vi "TestMove.vi"() -> ()   [LabVIEW 2017]
uses:
  <vilib>/userdefined/High Color/IMAQdx.ctl
  Global 5.vi
  <vilib>/vision/NI_Vision_Development_Module.lvlib
  <vilib>/vision/driver/NI_Vision_Acquisition_Software.lvlib
panel:
  out "x-y":dbl
  out "Back":bool
  out "ROI 2":T1
  out "Im3":T2(plugin-control)
  out "SecondCount":T2(plugin-control)
  out "Number of Objects 3":i32
  out "Less?":bool
  out "Encode Back":dbl
  out "Count Encode":dbl
  out "Status":string
  out "ROI":T1
  out "Count":T2(plugin-control)
  out "Extract":T2(plugin-control)
  out "Particle":T2(plugin-control)
  out "Threshold":T2(plugin-control)
  in  "Settings":T3={"Objects"=0, "Threshold"=128, "Reject Border"=FALSE, "Fill Holes"=FALSE, "Min Object Size"=FALSE, "Min Size"=3, "Max Object Size"=FALSE, "Max Size"=100, "Show Search Area"=FALSE, "Show Center"=TRUE, "Show Bounding Box"=TRUE} {"Objects" items=["Bright Objects", "Dark Objects"]; "Threshold" min=1 max=999999999 step=1; "Max Size" min=1 max=999999999 step=1; "Min Size" min=1 max=999999999 step=1}
  in  "Number of Objects":i32
  out "Number of Objects 2":i32
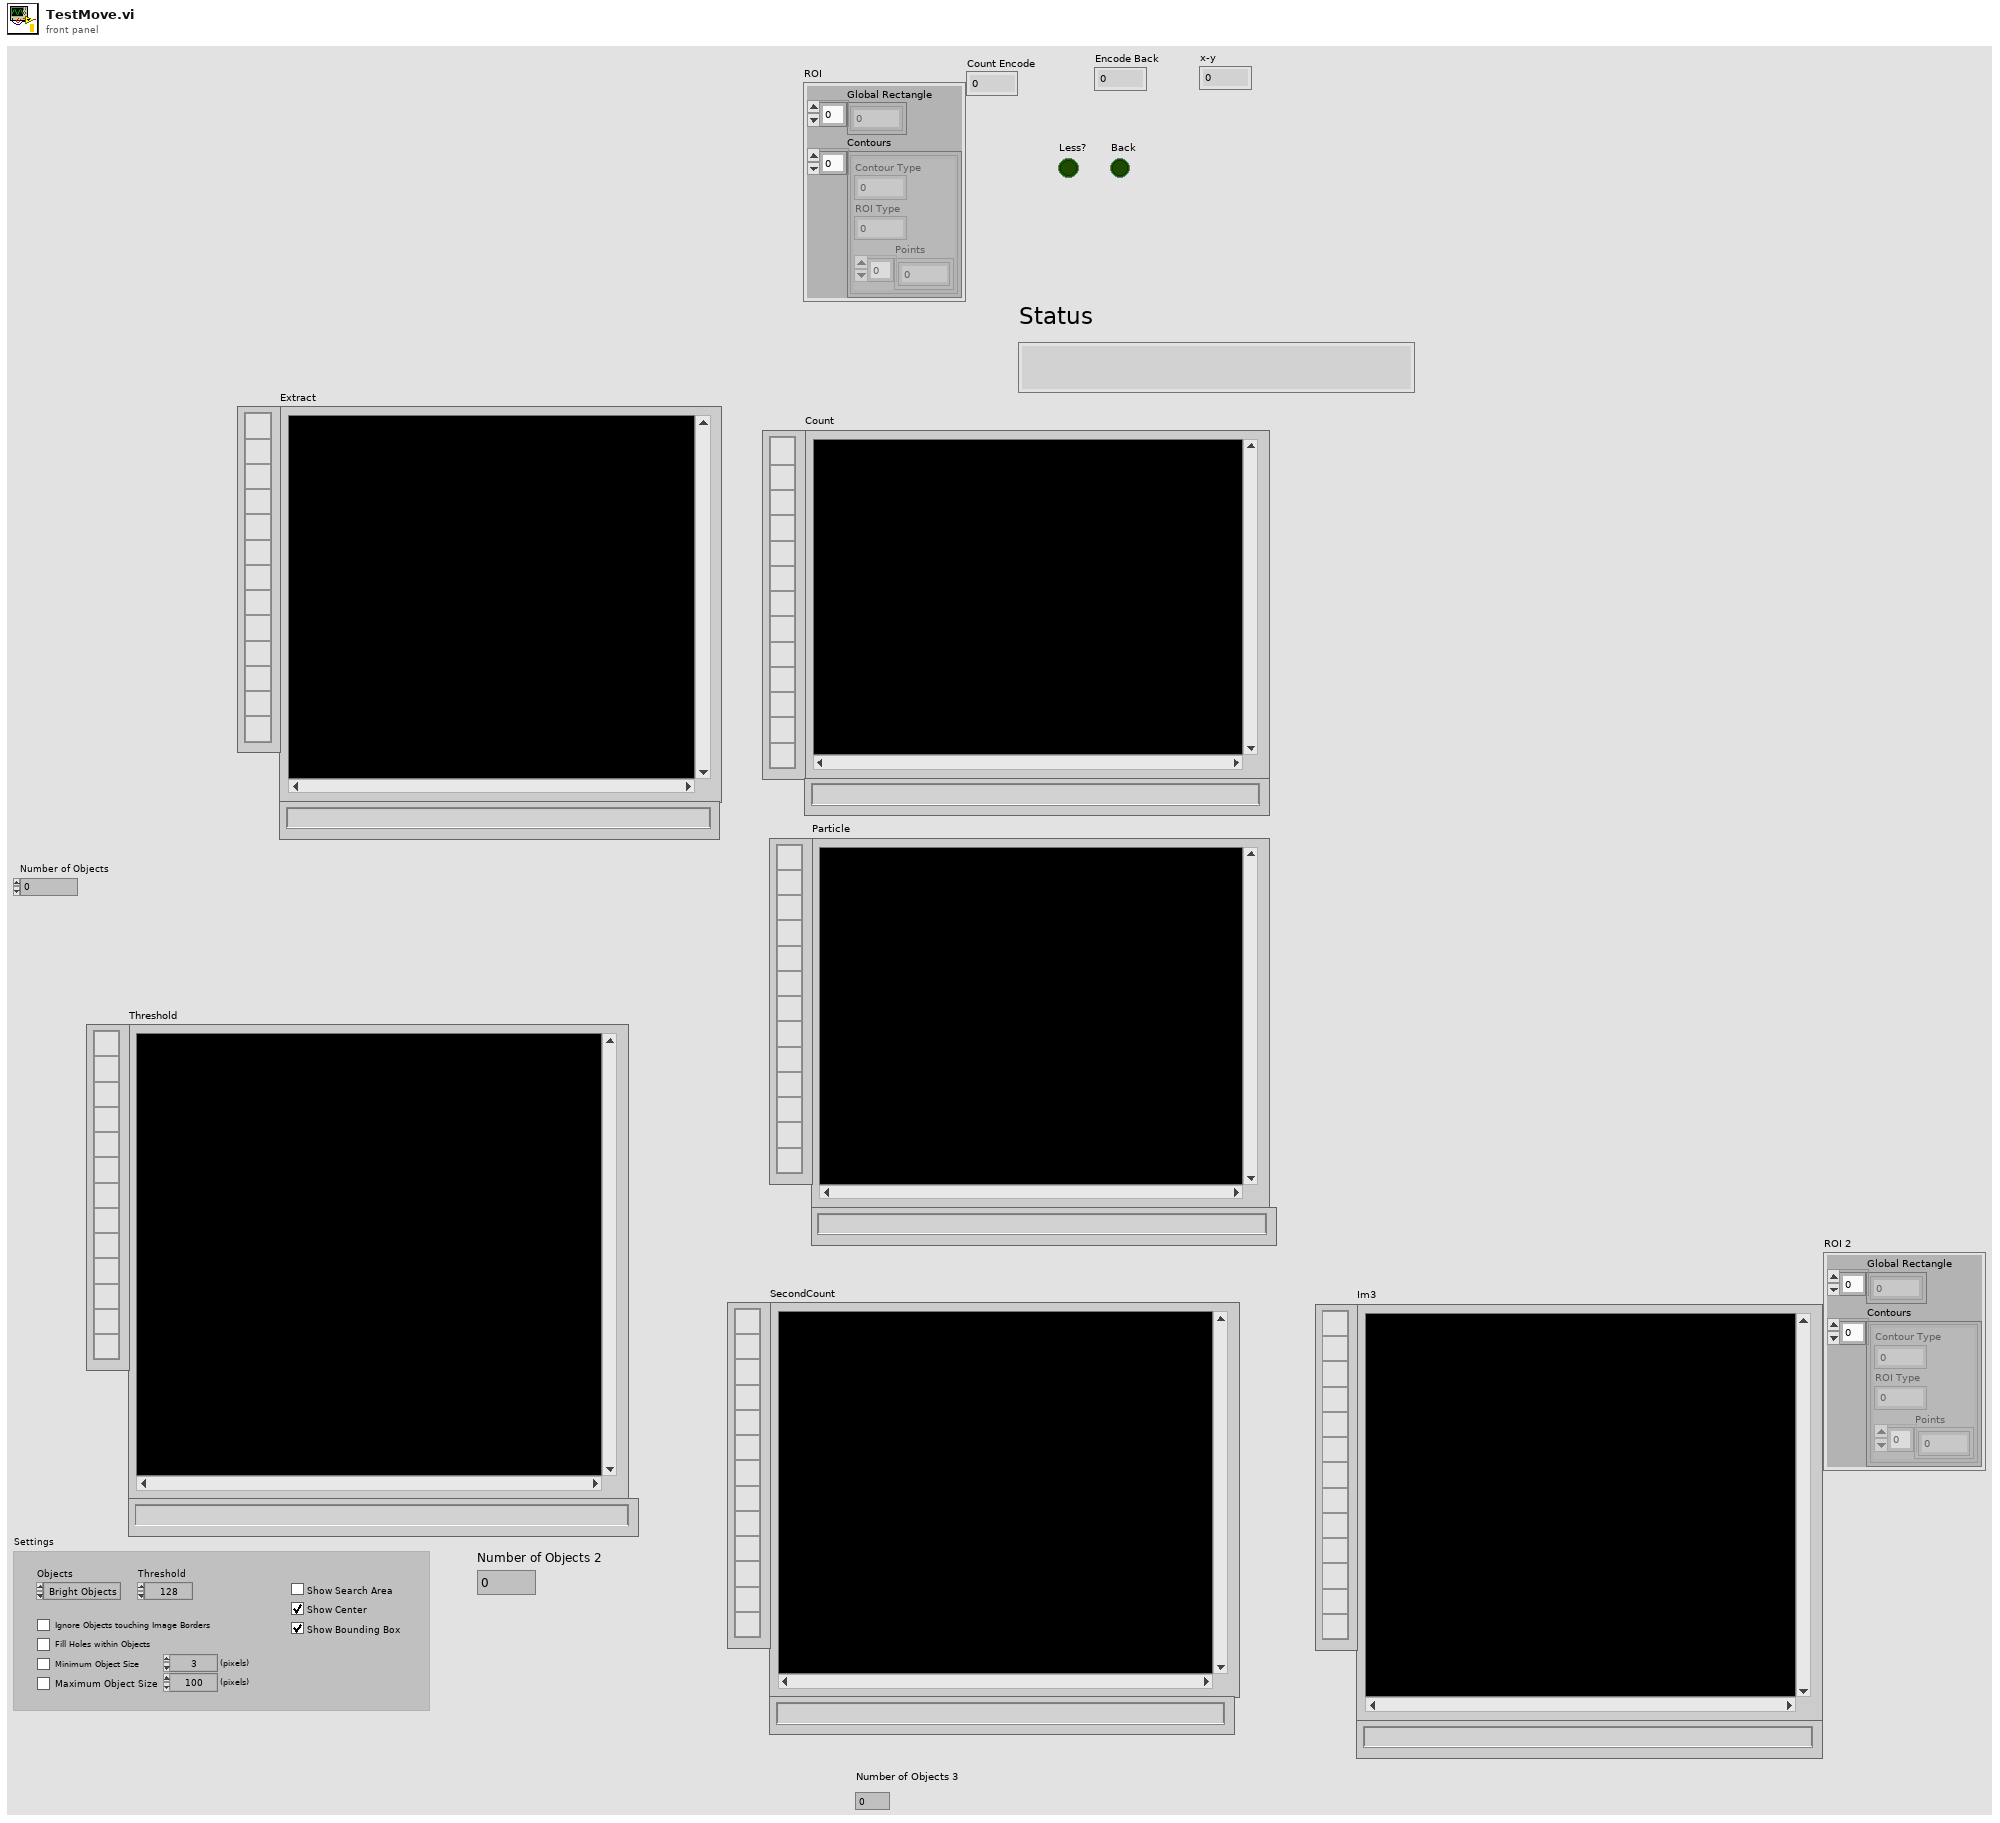
[diagram p1: front panel]
types:
  T1 = cluster{"Global Rectangle":i32[], "Contours":cluster{"Contour Type":u32, "ROI Type":u32, "Points":i32[]}[]}
  T2 = typedef "IMAQ Image.ctl" = refnum<image>
  T3 = cluster{"Objects":u16, "Threshold":i32, "Reject Border":bool, "Fill Holes":bool, "Min Object Size":bool, "Min Size":i32, "Max Object Size":bool, "Max Size":i32, "Show Search Area":bool, "Show Center":bool, "Show Bounding Box":bool}
  T4 = typedef "IMAQdx.ctl" = refnum<k21>
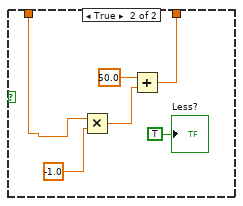
[diagram p2: hidden frame]
diagram:
  n1 = flat-sequence {
    tunnel: [w140] -> w90
    tunnel: [w139] -> w89
    tunnel: [w136] -> w88
    tunnel: [w151] -> w121
    tunnel: [w150] -> w120
    tunnel: w90 -> [w151]
    tunnel: w89 -> [w150]
    tunnel: w88 -> [w149]
    tunnel: [w148] -> w87
    tunnel: w121 -> [w160]
    tunnel: w120 -> [w159]
    tunnel: [w160] -> w115
    tunnel: [w159] -> w114
    tunnel: w87 -> [w158]
    tunnel: [w157] -> w86
    tunnel: [w170] -> w117
    tunnel: [w169] -> w116
    tunnel: w115 -> [w170]
    tunnel: w114 -> [w169]
    tunnel: w86 -> [w166]
    tunnel: [w164] -> w85
    tunnel: w117 -> [w179]
    tunnel: w116 -> [w178]
    tunnel: [w179] -> w103
    tunnel: [w178] -> w105
    tunnel: w85 -> [w177]
    tunnel: [w176] -> w83
    tunnel: w105 -> [w186]
    tunnel: [w186] -> w104
    tunnel: w103 -> [w185]
    tunnel: [w185] -> w102
    tunnel: [w183] -> w84
    tunnel: w83 -> [w183]
    tunnel: w104 -> [w193]
    tunnel: w102 -> [w192]
    tunnel: [w193] -> w119
    tunnel: [w192] -> w118
    tunnel: w84 -> [w189]
    tunnel: [w187] -> w82
    tunnel: w119 -> [w201]
    tunnel: w118 -> [w202]
    tunnel: [w202] -> w112
    tunnel: [w201] -> w110
    tunnel: w82 -> [w200]
    tunnel: [w199] -> w80
    tunnel: [w209] -> w113
    tunnel: w112 -> [w209]
    tunnel: [w208] -> w111
    tunnel: w110 -> [w208]
    tunnel: [w206] -> w81
    tunnel: w80 -> [w206]
    tunnel: [w212] -> w129
    tunnel: [w214] -> w128
    tunnel: w113 -> [w214]
    tunnel: w111 -> [w212]
    tunnel: w81 -> [w211]
    tunnel: [w210] -> w79
    tunnel: w129 -> [w223]
    tunnel: w128 -> [w224]
    tunnel: [w224] -> w109
    tunnel: [w223] -> w108
    tunnel: w79 -> [w222]
    tunnel: [w221] -> w78
    tunnel: [w232] -> w130
    tunnel: [w233] -> w127
    tunnel: w109 -> [w233]
    tunnel: w108 -> [w232]
    tunnel: w78 -> [w230]
    tunnel: [w228] -> w77
    tunnel: w130 -> [w240]
    tunnel: w127 -> [w241]
    tunnel: [w240] -> w56
    tunnel: w77 -> [w243]
    tunnel: [w242] -> w55
    tunnel: [w241] -> w54
    tunnel: [w240] -> w53
    tunnel: w56 -> [w253]
    tunnel: [w249] -> w107
    tunnel: [w253] -> w106
    tunnel: [w247] -> w76
    tunnel: w55 -> [w250]
    tunnel: w54 -> [w249]
    tunnel: w53 -> [w248]
    tunnel: [w308] -> w131
    tunnel: [w309] -> w126
    tunnel: w107 -> [w309]
    tunnel: w106 -> [w308]
    tunnel: w76 -> [w306]
    tunnel: [w304] -> w75
    tunnel: w131 -> [w319]
    tunnel: w126 -> [w318]
    tunnel: [w318] -> w101
    tunnel: [w319] -> w100
    tunnel: [w318] -> w99
    tunnel: w75 -> [w317]
    tunnel: [w316] -> w74
    tunnel: w101 -> [_]
    tunnel: w100 -> [w325]
    tunnel: [w325] -> w65
    tunnel: [w324] -> w64
    tunnel: w99 -> [w324]
    tunnel: w74 -> [w323]
    tunnel: [w323] -> w63
    tunnel: w65 -> [w331]
    tunnel: w64 -> [w332]
    tunnel: [w332] -> w94
    tunnel: [w331] -> w92
    tunnel: w63 -> [w329]
    tunnel: [w327] -> w73
    tunnel: w94 -> [w343]
    tunnel: [w343] -> w93
    tunnel: w92 -> [w344]
    tunnel: [w344] -> w91
    tunnel: w73 -> [w342]
    tunnel: [w341] -> w72
    tunnel: w93 -> [w356]
    tunnel: [w356] -> w98
    tunnel: w91 -> [w357]
    tunnel: [w357] -> w96
    tunnel: w72 -> [w354]
    tunnel: [w352] -> w71
    tunnel: w98 -> [w376]
    tunnel: [w376] -> w97
    tunnel: w96 -> [w375]
    tunnel: [w375] -> w95
    tunnel: w71 -> [w374]
    tunnel: [w373] -> w70
    tunnel: [w383] -> w125
    tunnel: [w384] -> w132
    tunnel: w97 -> [w384]
    tunnel: w95 -> [w383]
    tunnel: w70 -> [w382]
    tunnel: [w380] -> w69
    tunnel: w125 -> [w395]
    tunnel: [w395] -> w124
    tunnel: w132 -> [w394]
    tunnel: [w394] -> w133
    tunnel: w69 -> [w393]
    tunnel: [w392] -> w68
    tunnel: w124 -> [w403]
    tunnel: w133 -> [w404]
    tunnel: [w403] -> w123
    tunnel: [w404] -> w134
    tunnel: w68 -> [w401]
    tunnel: [w399] -> w67
    tunnel: w123 -> [w413]
    tunnel: w134 -> [w414]
    tunnel: [w414] -> w52
    tunnel: [w413] -> w50
    tunnel: w67 -> [w412]
    tunnel: [w411] -> w48
    tunnel: w52 -> [w420]
    tunnel: [w420] -> w51
    tunnel: w50 -> [w419]
    tunnel: [w419] -> w49
    tunnel: w48 -> [w418]
    tunnel: [w418] -> w47
    tunnel: [w426] -> w122
    tunnel: [w427] -> w135
    tunnel: w51 -> [w427]
    tunnel: w49 -> [w426]
    tunnel: w47 -> [w424]
    tunnel: [w422] -> w66
    tunnel: w122 -> [w432]
    tunnel: w135 -> [w433]
    tunnel: w66 -> [w435]
    tunnel: [w434] -> w44
    tunnel: [w433] -> w45
    tunnel: [w432] -> w46
    tunnel: [w442] -> w62
    tunnel: w46 -> [w442]
    tunnel: [w441] -> w61
    tunnel: w45 -> [w441]
    tunnel: [w440] -> w60
    tunnel: w44 -> [w440]
    tunnel: [w446] -> w59
    tunnel: w62 -> [w446]
    tunnel: [w445] -> w58
    tunnel: w61 -> [w445]
    tunnel: w60 -> [w449]
    tunnel: [w444] -> w57
    tunnel: w59 -> [w455]
    tunnel: w58 -> [w456]
    tunnel: w57 -> [w458]
    tunnel: [w457] -> w43
    tunnel: [w456] -> w42
    tunnel: [w455] -> w41
    tunnel: w43 -> [w465]
    tunnel: w42 -> [w463]
    tunnel: w41 -> [w462]
    tunnel: [w462] -> w40
    tunnel: [w464] -> w39
    tunnel: [w463] -> w37
    tunnel: [w462] -> w36
    tunnel: w40 -> [w479]
    tunnel: w39 -> [w478]
    tunnel: [w477] -> w38
    tunnel: w37 -> [w477]
    tunnel: w36 -> [w476]
    tunnel: [w476] -> w35
    tunnel: [w475] -> w31
    tunnel: w38 -> [w488]
    tunnel: w35 -> [w487]
    tunnel: [w486] -> w34
    tunnel: [w485] -> w33
    tunnel: [w484] -> w32
    tunnel: w31 -> [w483]
    tunnel: w34 -> [w540]
    tunnel: w33 -> [w538]
    tunnel: w32 -> [w537]
    tunnel: [w539] -> w30
    tunnel: [w538] -> w29
    tunnel: [w537] -> w28
    tunnel: w30 -> [w552]
    tunnel: w29 -> [w550]
    tunnel: w28 -> [w551]
    tunnel: [w551] -> w27
    tunnel: [w550] -> w25
    tunnel: [w549] -> w22
    tunnel: w27 -> [w559]
    tunnel: [w559] -> w26
    tunnel: w25 -> [w558]
    tunnel: [w558] -> w24
    tunnel: [w556] -> w23
    tunnel: w22 -> [w556]
    tunnel: w26 -> [w564]
    tunnel: w24 -> [w563]
    tunnel: w23 -> [w566]
    tunnel: [w562] -> w21
    tunnel: [w564] -> w20
    tunnel: [w563] -> w19
    tunnel: w21 -> [w577]
    tunnel: w20 -> [w576]
    tunnel: w19 -> [w575]
    tunnel: [w576] -> w18
    tunnel: [w575] -> w17
    tunnel: [w574] -> w16
    tunnel: w18 -> [w583]
    tunnel: w17 -> [w582]
    tunnel: w16 -> [w588]
    tunnel: [w584] -> w15
    tunnel: [w583] -> w13
    tunnel: [w582] -> w11
    tunnel: w15 -> [w597]
    tunnel: [w596] -> w14
    tunnel: w13 -> [w595]
    tunnel: [w595] -> w12
    tunnel: w11 -> [w594]
    tunnel: [w594] -> w10
    tunnel: w14 -> [w602]
    tunnel: w12 -> [w604]
    tunnel: w10 -> [w603]
    tunnel: [w604] -> w9
    tunnel: [w603] -> w7
    tunnel: [w602] -> w5
    tunnel: w9 -> [w615]
    tunnel: [w615] -> w8
    tunnel: w7 -> [w614]
    tunnel: [w614] -> w6
    tunnel: w5 -> [w613]
    tunnel: [w612] -> w4
    tunnel: w8 -> [w621]
    tunnel: w6 -> [w620]
    tunnel: w4 -> [w623]
    tunnel: [w621] -> w3
    tunnel: [w620] -> w2
    tunnel: [w619] -> w1
    tunnel: w3 -> [w633]
    tunnel: w2 -> [w632]
    tunnel: w1 -> [w631]
    frame #0 {
      w140 = tag "B/I2C" ("myRIO MXP Port A/B")
      w139 = u8 1 ("Controller ID#  (I2C Address)")
      # "enable"
      n2 = Wait (ms)(milliseconds to wait=u32 1000) -> ()  [unwired: 1 out]
      n3 = local write "Status"("Starting" ("Status")) -> ()
      n4 = call <vilib>:"TETRIX_Enable_DC_Controller_myRIO.vi"("myRIO MXP Port A/B"=w140, "Controller ID#  (I2C Address)"=w139) -> ("Error/Flow Out"=w138:errorcluster)  [unwired: 5 in]
      n5 = call <vilib>:"TETRIX_Motor_Invert_myRIO.vi"("myRIO MXP Port A/B"=w140, "Invert State"=TRUE, "Select Channel"="Motor 1", "Controller ID#  (I2C Address)"=w139) -> ()  [unwired: 3 in, 1 out]
      n6 = call <vilib>:"TETRIX_Reset_Encoders_myRIO.vi"("myRIO MXP Port A/B"=w140, "Select Encoder"="Encoders 1 and 2", "Controller ID#  (I2C Address)"=w139, "Error/Flow In"=w138) -> ("Error/Flow Out"=w137:errorcluster)  [unwired: 3 in]
      n7 = call <vilib>:"TETRIX_Stop_Motors_myRIO.vi"("myRIO MXP Port A/B"=w140, "Stop Mode"="Brake", "Select Channel"="Both Motors", "Controller ID#  (I2C Address)"=w139, "Error/Flow In"=w137) -> ("Error/Flow Out"=w136:errorcluster)  [unwired: 2 in]
    }
    frame #1 {
      w153 = 660 ("Motor 2 Encoder Target")
      w155 = i16 200 ("Motor 1 Contant Speed (Degrees per Second)")
      # "fate 1 start position"
      n8 = Wait (ms)(milliseconds to wait=u32 5500) -> ()  [unwired: 1 out]
      n9 = call <vilib>:"TETRIX_Set_Motor_Target(s)_myRIO.vi"("Motor 2 Encoder Target"=w153, "Motor 1 Encoder Target"=w153, "myRIO MXP Port A/B"=w151, "Controller ID#  (I2C Address)"=w150, "Motor 2 Constant Speed (Degrees per Second)"=w155, "Motor 1 Contant Speed (Degrees per Second)"=w155, "Encoder Units"="Degrees", "Error/Flow In"=w149) -> ("Error/Flow Out"=w148:errorcluster)  [unwired: 1 in]
      "Status" <- "Phase 1" ("Status")
    }
    frame #2 {
      n10 = Wait (ms)(milliseconds to wait=u32 500) -> ()  [unwired: 1 out]
      n11 = call <vilib>:"TETRIX_Stop_Motors_myRIO.vi"("myRIO MXP Port A/B"=w160, "Stop Mode"="Brake", "Select Channel"="Both Motors", "Controller ID#  (I2C Address)"=w159, "Error/Flow In"=w158) -> ("Error/Flow Out"=w157:errorcluster)  [unwired: 2 in]
    }
    frame #3 {
      w175 = i16 100 ("Motor 1 Contant Speed (Degrees per Second)")
      # "fate 2 catch ball"
      n12 = Wait (ms)(milliseconds to wait=u32 3000) -> ()  [unwired: 1 out]
      n13 = local write "Status"("Turning" ("Status")) -> ()
      n14 = call <vilib>:"TETRIX_Reset_Encoders_myRIO.vi"("myRIO MXP Port A/B"=w170, "Select Encoder"="Encoders 1 and 2", "Controller ID#  (I2C Address)"=w169, "Error/Flow In"=w166) -> ("Error/Flow Out"=w165:errorcluster)  [unwired: 3 in]
      n15 = call <vilib>:"TETRIX_Set_Motor_Target(s)_myRIO.vi"("Motor 2 Encoder Target"=300 ("Motor 1 Encoder Target"), "Motor 1 Encoder Target"=-290, "myRIO MXP Port A/B"=w170, "Controller ID#  (I2C Address)"=w169, "Motor 2 Constant Speed (Degrees per Second)"=w175, "Motor 1 Contant Speed (Degrees per Second)"=w175, "Encoder Units"="Degrees", "Error/Flow In"=w165) -> ("Error/Flow Out"=w164:errorcluster)  [unwired: 1 in]
    }
    frame #4 {
      n16 = Wait (ms)(milliseconds to wait=u32 500) -> ()  [unwired: 1 out]
      n17 = call <vilib>:"TETRIX_Stop_Motors_myRIO.vi"("myRIO MXP Port A/B"=w179, "Stop Mode"="Brake", "Select Channel"="Both Motors", "Controller ID#  (I2C Address)"=w178, "Error/Flow In"=w177) -> ("Error/Flow Out"=w176:errorcluster)  [unwired: 2 in]
    }
    frame #5 {
      n18 = local write "Status"("Move Gripper" ("Status")) -> ()
      n19 = call "ServoPickup.vi"() -> ()  [unwired: 12 in]
    }
    frame #6 {
      w195 = i16 100 ("Motor 1 Contant Speed (Degrees per Second)")
      n20 = Wait (ms)(milliseconds to wait=u32 5000) -> ()  [unwired: 1 out]
      n21 = local write "Status"("Moving to catch" ("Status")) -> ()
      n22 = call <vilib>:"TETRIX_Reset_Encoders_myRIO.vi"("myRIO MXP Port A/B"=w192, "Select Encoder"="Encoders 1 and 2", "Controller ID#  (I2C Address)"=w193, "Error/Flow In"=w189) -> ("Error/Flow Out"=w188:errorcluster)  [unwired: 3 in]
      n23 = call <vilib>:"TETRIX_Set_Motor_Target(s)_myRIO.vi"("Motor 2 Encoder Target"=390 ("Motor 1 Encoder Target"), "Motor 1 Encoder Target"=390, "myRIO MXP Port A/B"=w192, "Controller ID#  (I2C Address)"=w193, "Motor 2 Constant Speed (Degrees per Second)"=w195, "Motor 1 Contant Speed (Degrees per Second)"=w195, "Encoder Units"="Degrees", "Error/Flow In"=w188) -> ("Error/Flow Out"=w187:errorcluster)  [unwired: 1 in]
    }
    frame #7 {
      n24 = Wait (ms)(milliseconds to wait=u32 500) -> ()  [unwired: 1 out]
      n25 = call <vilib>:"TETRIX_Stop_Motors_myRIO.vi"("myRIO MXP Port A/B"=w202, "Stop Mode"="Brake", "Select Channel"="Both Motors", "Controller ID#  (I2C Address)"=w201, "Error/Flow In"=w200) -> ("Error/Flow Out"=w199:errorcluster)  [unwired: 2 in]
    }
    frame #8 {
      n26 = local write "Status"("Catching" ("Status")) -> ()
      n27 = call "PickBall.vi"() -> ()  [unwired: 12 in]
    }
    frame #9 {
      w217 = i16 100 ("Motor 1 Contant Speed (Degrees per Second)")
      n28 = Wait (ms)(milliseconds to wait=u32 4200) -> ()  [unwired: 1 out]
      n29 = call <vilib>:"TETRIX_Set_Motor_Target(s)_myRIO.vi"("Motor 2 Encoder Target"=390 ("Motor 1 Encoder Target"), "Motor 1 Encoder Target"=390, "myRIO MXP Port A/B"=w214, "Controller ID#  (I2C Address)"=w212, "Motor 2 Constant Speed (Degrees per Second)"=w217, "Motor 1 Contant Speed (Degrees per Second)"=w217, "Encoder Units"="Degrees", "Error/Flow In"=w211) -> ("Error/Flow Out"=w210:errorcluster)  [unwired: 1 in]
      n30 = local write "Status"("Moving to Bowling" ("Status")) -> ()
      n31 = call <vilib>:"TETRIX_Reset_Encoders_myRIO.vi"("myRIO MXP Port A/B"=w214, "Select Encoder"="Encoders 1 and 2", "Controller ID#  (I2C Address)"=w212) -> ()  [unwired: 4 in, 1 out]
    }
    frame #10 {
      # "end fate2"
      n32 = Wait (ms)(milliseconds to wait=u32 500) -> ()  [unwired: 1 out]
      n33 = call <vilib>:"TETRIX_Stop_Motors_myRIO.vi"("myRIO MXP Port A/B"=w224, "Stop Mode"="Brake", "Select Channel"="Both Motors", "Controller ID#  (I2C Address)"=w223, "Error/Flow In"=w222) -> ("Error/Flow Out"=w221:errorcluster)  [unwired: 2 in]
    }
    frame #11 {
      w237 = i16 100 ("Motor 2 Constant Speed (Degrees per Second)")
      # "fate 3  go to shoot ball position"
      n34 = Wait (ms)(milliseconds to wait=u32 3000) -> ()  [unwired: 1 out]
      n35 = local write "Status"("Phase 3 Turning" ("Status")) -> ()
      n36 = call <vilib>:"TETRIX_Reset_Encoders_myRIO.vi"("myRIO MXP Port A/B"=w233, "Select Encoder"="Encoders 1 and 2", "Controller ID#  (I2C Address)"=w232, "Error/Flow In"=w230) -> ("Error/Flow Out"=w229:errorcluster)  [unwired: 3 in]
      n37 = call <vilib>:"TETRIX_Set_Motor_Target(s)_myRIO.vi"("Motor 2 Encoder Target"=300, "Motor 1 Encoder Target"=-295, "myRIO MXP Port A/B"=w233, "Controller ID#  (I2C Address)"=w232, "Motor 2 Constant Speed (Degrees per Second)"=w237, "Motor 1 Contant Speed (Degrees per Second)"=w237, "Encoder Units"="Degrees", "Error/Flow In"=w229) -> ("Error/Flow Out"=w228:errorcluster)  [unwired: 1 in]
    }
    frame #12 {
      n38 = Wait (ms)(milliseconds to wait=u32 500) -> ()  [unwired: 1 out]
      n39 = call <vilib>:"TETRIX_Stop_Motors_myRIO.vi"("myRIO MXP Port A/B"=w241, "Stop Mode"="Brake", "Select Channel"="Both Motors", "Controller ID#  (I2C Address)"=w240, "Error/Flow In"=w243) -> ("Error/Flow Out"=w242:errorcluster)  [unwired: 2 in]
    }
    frame #13 {
      (unwired) "im0" ("Image Name")
      n40 = global write "Global 5.vi" "Count Encode"(0.0 ("Count Encode")) -> ()
      n41 = call "IMAQ Create"("Image Name"="im0") -> ("New Image"=w256:T2)  [unwired: 4 in, 1 out]
      n42 = call "IMAQ Create"("Image Name"="im1") -> ("New Image"=w254:T2)  [unwired: 4 in, 1 out]
      n43 = while {
        tunnel: w256 -> [w282]
        tunnel: w254 -> [w279]
        tunnel: w249 -> [w274]
        tunnel: w248 -> [w275]
        tunnel: w250 -> [w262]
        tunnel: w249 -> [w260]
        tunnel: w248 -> [w259]
        tunnel: [w258] -> w247
        stop <- w272 stop-if-true
        w283 = u16 1 items=["RGB", "HSL", "HSV", "HSI"] ("Color Mode")
        n44 = flat-sequence {
          tunnel: w275 -> [w296]
          tunnel: w274 -> [w295]
          tunnel: w262 -> [w287]
          tunnel: [w285] -> w261
          tunnel: w261 -> [w298]
          tunnel: w260 -> [w302]
          tunnel: w259 -> [w299]
          tunnel: [w297] -> w258
          frame #0 {
            w288 = 50 ("Motor 1 Encoder Target")
            w292 = i16 100 ("Motor 1 Contant Speed (Degrees per Second)")
            n45 = global read "Global 5.vi" "Count Encode"() -> (w289:dbl)
            n46 = Wait (ms)(milliseconds to wait=u32 500 ("millisecond timer value")) -> ()  [unwired: 1 out]
            n47 = Add(x=w288, y=w289) -> (x+y=w290:dbl)
            n48 = call <vilib>:"TETRIX_Reset_Encoders_myRIO.vi"("myRIO MXP Port A/B"=w295, "Select Encoder"="Encoders 1 and 2", "Controller ID#  (I2C Address)"=w296, "Error/Flow In"=w287) -> ("Error/Flow Out"=w286:errorcluster)  [unwired: 3 in]
            n49 = call <vilib>:"TETRIX_Set_Motor_Target(s)_myRIO.vi"("Motor 2 Encoder Target"=w288, "Motor 1 Encoder Target"=w288, "myRIO MXP Port A/B"=w295, "Motor 2 Constant Speed (Degrees per Second)"=w292, "Motor 1 Contant Speed (Degrees per Second)"=w292, "Encoder Units"="Degrees", "Error/Flow In"=w286) -> ("Error/Flow Out"=w285:errorcluster)  [unwired: 2 in]
            n50 = global write "Global 5.vi" "Count Encode"(w290) -> ()
          }
          frame #1 {
            n51 = Wait (ms)(milliseconds to wait=u32 500 ("millisecond timer value")) -> ()  [unwired: 1 out]
            n52 = call <vilib>:"TETRIX_Stop_Motors_myRIO.vi"("myRIO MXP Port A/B"=w302, "Stop Mode"="Brake", "Select Channel"="Both Motors", "Controller ID#  (I2C Address)"=w299, "Error/Flow In"=w298) -> ("Error/Flow Out"=w297:errorcluster)  [unwired: 2 in]
          }
        }
        n53 = property on="Count" class="ImageControl"() -> ("ROI"=→"ROI":T1)  [unwired: 2 in, 2 out]
        n54 = call <vilib>:"IMAQdx Snap2.vi"("Image In"=w282, "Session In"=T4 "cam0") -> ("Image Out"=w284:T2)  [unwired: 7 in, 2 out]
        n55 = call "IMAQ ExtractColorPlanes"("Blue or Luma or Val or Inten Plane"=w279, "Color Mode"=w283, "Image Src"=w284) -> ("Blue or Luma or Val or Inten Plane out"=w280:T2)  [unwired: 5 in, 3 out]
        n56 = call "IMAQ Rotate"("Angle (degrees)"=sgl -1.5, "Image Src"=w280) -> ("Image Dst Out"=w268:T2)  [unwired: 8 in, 1 out]
        "Count" <- w268
        n57 = call "IMAQ Extract 2"("Optional Rectangle"=i32[] [321, 232, 340, 263], "Image Src"=w268) -> ("Image Dst Out"=w278:T2)  [unwired: 8 in, 1 out]
        "Extract" <- w278
        "Particle" <- w278
        n58 = global read "Global 5.vi" "Count Encode"() -> (w271:dbl)
        "Count Encode" <- w271
        n59 = call "IMAQ Count Objects 2"("Settings"="Settings", "Image"=w278) -> ("Number of Objects"=w265:i32, "Image Out"=→"Threshold":T2)  [unwired: 5 in, 3 out]
        "Number of Objects 2" <- w265
        n60 = Greater?(x=w265, y=2) -> (0:w266:bool)
        n61 = Greater Or Equal?(x=w271, y=840.0) -> (x >= y?=w269:bool)
        n62 = Or(x=w266, y=w269) -> (x .or. y?=w272:bool)
      }
      n63 = local write "Status"("IMAQ Start" ("Status")) -> ()
    }
    frame #14 {
      w314 = i16 100 ("Motor 1 Contant Speed (Degrees per Second)")
      n64 = Wait (ms)(milliseconds to wait=u32 3000) -> ()  [unwired: 1 out]
      n65 = local write "Status"("Turning to shoot" ("Status")) -> ()
      n66 = call <vilib>:"TETRIX_Reset_Encoders_myRIO.vi"("myRIO MXP Port A/B"=w309, "Select Encoder"="Encoders 1 and 2", "Controller ID#  (I2C Address)"=w308, "Error/Flow In"=w306) -> ("Error/Flow Out"=w305:errorcluster)  [unwired: 3 in]
      n67 = call <vilib>:"TETRIX_Set_Motor_Target(s)_myRIO.vi"("Motor 2 Encoder Target"=-285, "Motor 1 Encoder Target"=290, "myRIO MXP Port A/B"=w309, "Controller ID#  (I2C Address)"=w308, "Motor 2 Constant Speed (Degrees per Second)"=w314, "Motor 1 Contant Speed (Degrees per Second)"=w314, "Encoder Units"="Degrees", "Error/Flow In"=w305) -> ("Error/Flow Out"=w304:errorcluster)  [unwired: 1 in]
    }
    frame #15 {
      n68 = Wait (ms)(milliseconds to wait=u32 500) -> ()  [unwired: 1 out]
      n69 = call <vilib>:"TETRIX_Stop_Motors_myRIO.vi"("myRIO MXP Port A/B"=w318, "Stop Mode"="Brake", "Select Channel"="Both Motors", "Controller ID#  (I2C Address)"=w319, "Error/Flow In"=w317) -> ("Error/Flow Out"=w316:errorcluster)  [unwired: 2 in]
    }
    frame #16 {
      # "fate 4 shoot ball"
      n70 = local write "Status"(" Shooting" ("Status")) -> ()
      n71 = call "Shoot.vi"() -> ()  [unwired: 12 in]
    }
    frame #17 {
      w337 = i16 100 ("Motor 1 Contant Speed (Degrees per Second)")
      n72 = Wait (ms)(milliseconds to wait=u32 3000) -> ()  [unwired: 1 out]
      n73 = local write "Status"("Turning to Check" ("Status")) -> ()
      n74 = call <vilib>:"TETRIX_Reset_Encoders_myRIO.vi"("myRIO MXP Port A/B"=w332, "Select Encoder"="Encoders 1 and 2", "Controller ID#  (I2C Address)"=w331, "Error/Flow In"=w329) -> ("Error/Flow Out"=w328:errorcluster)  [unwired: 3 in]
      n75 = call <vilib>:"TETRIX_Set_Motor_Target(s)_myRIO.vi"("Motor 2 Encoder Target"=300, "Motor 1 Encoder Target"=-285, "myRIO MXP Port A/B"=w332, "Controller ID#  (I2C Address)"=w331, "Motor 2 Constant Speed (Degrees per Second)"=w337, "Motor 1 Contant Speed (Degrees per Second)"=w337, "Encoder Units"="Degrees", "Error/Flow In"=w328) -> ("Error/Flow Out"=w327:errorcluster)  [unwired: 1 in]
    }
    frame #18 {
      n76 = Wait (ms)(milliseconds to wait=u32 500) -> ()  [unwired: 1 out]
      n77 = local write "Less?"(FALSE ("Less?")) -> ()
      n78 = local write "Encode Back"(0.0 ("Encode Back")) -> ()
      n79 = call <vilib>:"TETRIX_Stop_Motors_myRIO.vi"("myRIO MXP Port A/B"=w343, "Stop Mode"="Brake", "Select Channel"="Both Motors", "Controller ID#  (I2C Address)"=w344, "Error/Flow In"=w342) -> ("Error/Flow Out"=w341:errorcluster)  [unwired: 2 in]
    }
    frame #19 {
      w360 = i16 200 ("Motor 1 Contant Speed (Degrees per Second)")
      n80 = global read "Global 5.vi" "Count Encode"() -> (w349:dbl)
      n81 = Wait (ms)(milliseconds to wait=u32 5000) -> ()  [unwired: 1 out]
      n82 = local write "Status"("Backwarding" ("Status")) -> ()
      n83 = call <vilib>:"TETRIX_Reset_Encoders_myRIO.vi"("myRIO MXP Port A/B"=w356, "Select Encoder"="Encoders 1 and 2", "Controller ID#  (I2C Address)"=w357, "Error/Flow In"=w354) -> ("Error/Flow Out"=w353:errorcluster)  [unwired: 3 in]
      n84 = Less Or Equal?(x=w349, y=100.0) -> (x <= y?=w351:bool)
      n85 = case shown="False" w351 {
        tunnel: [w363 w368] -> w350
        tunnel: w349 -> [w362 w371]
        frame False {
          n86 = Multiply(x=-1.0, y=w362) -> (x*y=w366:dbl)
          n87 = Add(x=85.0, y=w366) -> (x+y=w363:dbl)
        }
        frame True {
          n88 = Multiply(x=w371, y=-1.0) -> (x*y=w369:dbl)
          n89 = Add(x=50.0, y=w369) -> (x+y=w368:dbl)
          "Less?" <- TRUE ("Less?")
        }
      }
      "Encode Back" <- w350
      n90 = call <vilib>:"TETRIX_Set_Motor_Target(s)_myRIO.vi"("Motor 2 Encoder Target"=w350, "Motor 1 Encoder Target"=w350, "myRIO MXP Port A/B"=w356, "Controller ID#  (I2C Address)"=w357, "Motor 2 Constant Speed (Degrees per Second)"=w360, "Motor 1 Contant Speed (Degrees per Second)"=w360, "Encoder Units"="Degrees", "Error/Flow In"=w353) -> ("Error/Flow Out"=w352:errorcluster)  [unwired: 1 in]
    }
    frame #20 {
      n91 = Wait (ms)(milliseconds to wait=u32 500) -> ()  [unwired: 1 out]
      n92 = call <vilib>:"TETRIX_Stop_Motors_myRIO.vi"("myRIO MXP Port A/B"=w376, "Stop Mode"="Brake", "Select Channel"="Both Motors", "Controller ID#  (I2C Address)"=w375, "Error/Flow In"=w374) -> ("Error/Flow Out"=w373:errorcluster)  [unwired: 2 in]
    }
    frame #21 {
      w390 = i16 100 ("Motor 1 Contant Speed (Degrees per Second)")
      # "fate 5 go home"
      n93 = Wait (ms)(milliseconds to wait=u32 3000) -> ()  [unwired: 1 out]
      n94 = call <vilib>:"TETRIX_Reset_Encoders_myRIO.vi"("myRIO MXP Port A/B"=w384, "Select Encoder"="Encoders 1 and 2", "Controller ID#  (I2C Address)"=w383, "Error/Flow In"=w382) -> ("Error/Flow Out"=w381:errorcluster)  [unwired: 3 in]
      n95 = local write "Status"("Turning to rack" ("Status")) -> ()
      n96 = call <vilib>:"TETRIX_Set_Motor_Target(s)_myRIO.vi"("Motor 2 Encoder Target"=-285, "Motor 1 Encoder Target"=290, "Controller ID#  (I2C Address)"=w383, "Motor 2 Constant Speed (Degrees per Second)"=w390, "Motor 1 Contant Speed (Degrees per Second)"=w390, "Encoder Units"="Degrees", "Error/Flow In"=w381) -> ("Error/Flow Out"=w380:errorcluster)  [unwired: 2 in]
    }
    frame #22 {
      n97 = Wait (ms)(milliseconds to wait=u32 500) -> ()  [unwired: 1 out]
      n98 = call <vilib>:"TETRIX_Stop_Motors_myRIO.vi"("myRIO MXP Port A/B"=w394, "Stop Mode"="Brake", "Select Channel"="Both Motors", "Controller ID#  (I2C Address)"=w395, "Error/Flow In"=w393) -> ("Error/Flow Out"=w392:errorcluster)  [unwired: 2 in]
    }
    frame #23 {
      w409 = i16 150 ("Motor 1 Contant Speed (Degrees per Second)")
      n99 = Wait (ms)(milliseconds to wait=u32 5000) -> ()  [unwired: 1 out]
      n100 = local write "Status"("backwarding to rack " ("Status")) -> ()
      n101 = call <vilib>:"TETRIX_Reset_Encoders_myRIO.vi"("myRIO MXP Port A/B"=w404, "Select Encoder"="Encoders 1 and 2", "Controller ID#  (I2C Address)"=w403, "Error/Flow In"=w401) -> ("Error/Flow Out"=w400:errorcluster)  [unwired: 3 in]
      n102 = call <vilib>:"TETRIX_Set_Motor_Target(s)_myRIO.vi"("Motor 2 Encoder Target"=-400 ("Motor 1 Encoder Target"), "Motor 1 Encoder Target"=-400, "myRIO MXP Port A/B"=w404, "Controller ID#  (I2C Address)"=w403, "Motor 2 Constant Speed (Degrees per Second)"=w409, "Motor 1 Contant Speed (Degrees per Second)"=w409, "Encoder Units"="Degrees", "Error/Flow In"=w400) -> ("Error/Flow Out"=w399:errorcluster)  [unwired: 1 in]
    }
    frame #24 {
      n103 = Wait (ms)(milliseconds to wait=u32 500) -> ()  [unwired: 1 out]
      n104 = call <vilib>:"TETRIX_Stop_Motors_myRIO.vi"("myRIO MXP Port A/B"=w414, "Stop Mode"="Brake", "Select Channel"="Both Motors", "Controller ID#  (I2C Address)"=w413, "Error/Flow In"=w412) -> ("Error/Flow Out"=w411:errorcluster)  [unwired: 2 in]
    }
    frame #25 {
      n105 = call "ServoPickup.vi"() -> ()  [unwired: 12 in]
    }
    frame #26 {
      w421 = 70 ("Motor 1 Encoder Target")
      w431 = i16 100 ("Motor 1 Contant Speed (Degrees per Second)")
      n106 = Wait (ms)(milliseconds to wait=u32 5000) -> ()  [unwired: 1 out]
      n107 = local write "Status"("Go to Rack " ("Status")) -> ()
      n108 = call <vilib>:"TETRIX_Reset_Encoders_myRIO.vi"("myRIO MXP Port A/B"=w427, "Select Encoder"="Encoders 1 and 2", "Controller ID#  (I2C Address)"=w426, "Error/Flow In"=w424) -> ("Error/Flow Out"=w423:errorcluster)  [unwired: 3 in]
      n109 = call <vilib>:"TETRIX_Set_Motor_Target(s)_myRIO.vi"("Motor 2 Encoder Target"=w421, "Motor 1 Encoder Target"=w421, "myRIO MXP Port A/B"=w427, "Controller ID#  (I2C Address)"=w426, "Motor 2 Constant Speed (Degrees per Second)"=w431, "Motor 1 Contant Speed (Degrees per Second)"=w431, "Encoder Units"="Degrees", "Error/Flow In"=w423) -> ("Error/Flow Out"=w422:errorcluster)  [unwired: 1 in]
    }
    frame #27 {
      n110 = Wait (ms)(milliseconds to wait=u32 500) -> ()  [unwired: 1 out]
      n111 = call <vilib>:"TETRIX_Stop_Motors_myRIO.vi"("myRIO MXP Port A/B"=w433, "Stop Mode"="Brake", "Select Channel"="Both Motors", "Controller ID#  (I2C Address)"=w432, "Error/Flow In"=w435) -> ("Error/Flow Out"=w434:errorcluster)  [unwired: 2 in]
    }
    frame #28 {
      n112 = call "PickBall.vi"() -> ()  [unwired: 12 in]
      n113 = local write "Status"(" Catching ball" ("Status")) -> ()
    }
    frame #29 {
      w454 = i16 200 ("Motor 1 Contant Speed (Degrees per Second)")
      n114 = Wait (ms)(milliseconds to wait=u32 4500) -> ()  [unwired: 1 out]
      n115 = call <vilib>:"TETRIX_Reset_Encoders_myRIO.vi"("myRIO MXP Port A/B"=w445, "Select Encoder"="Encoders 1 and 2", "Controller ID#  (I2C Address)"=w446, "Error/Flow In"=w449) -> ("Error/Flow Out"=w448:errorcluster)  [unwired: 3 in]
      n116 = local write "Status"("Move to Shoot " ("Status")) -> ()
      n117 = call <vilib>:"TETRIX_Set_Motor_Target(s)_myRIO.vi"("Motor 2 Encoder Target"=300 ("Motor 1 Encoder Target"), "Motor 1 Encoder Target"=300, "myRIO MXP Port A/B"=w445, "Controller ID#  (I2C Address)"=w446, "Motor 2 Constant Speed (Degrees per Second)"=w454, "Motor 1 Contant Speed (Degrees per Second)"=w454, "Encoder Units"="Degrees", "Error/Flow In"=w448) -> ("Error/Flow Out"=w444:errorcluster)  [unwired: 1 in]
    }
    frame #30 {
      n118 = call <vilib>:"TETRIX_Stop_Motors_myRIO.vi"("myRIO MXP Port A/B"=w456, "Stop Mode"="Brake", "Select Channel"="Both Motors", "Controller ID#  (I2C Address)"=w455, "Error/Flow In"=w458) -> ("Error/Flow Out"=w457:errorcluster)  [unwired: 2 in]
    }
    frame #31 {
      w466 = i16 200 ("Motor 1 Contant Speed (Degrees per Second)")
      n119 = Wait (ms)(milliseconds to wait=u32 4500) -> ()  [unwired: 1 out]
      n120 = local write "Status"("Turning  " ("Status")) -> ()
      n121 = call <vilib>:"TETRIX_Reset_Encoders_myRIO.vi"("myRIO MXP Port A/B"=w463, "Select Encoder"="Encoders 1 and 2", "Controller ID#  (I2C Address)"=w462, "Error/Flow In"=w465) -> ("Error/Flow Out"=w471:errorcluster)  [unwired: 3 in]
      n122 = call <vilib>:"TETRIX_Set_Motor_Target(s)_myRIO.vi"("Motor 2 Encoder Target"=300 ("Motor 1 Encoder Target"), "Motor 1 Encoder Target"=-295, "myRIO MXP Port A/B"=w463, "Controller ID#  (I2C Address)"=w462, "Motor 2 Constant Speed (Degrees per Second)"=w466, "Motor 1 Contant Speed (Degrees per Second)"=w466, "Encoder Units"="Degrees", "Error/Flow In"=w471) -> ("Error/Flow Out"=w464:errorcluster)  [unwired: 1 in]
    }
    frame #32 {
      n123 = global write "Global 5.vi" "Count Encode"(0.0 ("Count Encode")) -> ()
      n124 = Wait (ms)(milliseconds to wait=u32 500) -> ()  [unwired: 1 out]
      n125 = call <vilib>:"TETRIX_Stop_Motors_myRIO.vi"("myRIO MXP Port A/B"=w477, "Stop Mode"="Brake", "Select Channel"="Both Motors", "Controller ID#  (I2C Address)"=w479, "Error/Flow In"=w478) -> ("Error/Flow Out"=w475:errorcluster)  [unwired: 2 in]
    }
    frame #33 {
      n126 = call "IMAQ Create"("Image Name"="im5") -> ("New Image"=w491:T2)  [unwired: 4 in, 1 out]
      n127 = call "IMAQ Create"("Image Name"="im7") -> ("New Image"=w492:T2)  [unwired: 4 in, 1 out]
      n128 = while {
        tunnel: w492 -> [w517]
        tunnel: w491 -> [w511]
        tunnel: w488 -> [w500]
        tunnel: w487 -> [w499]
        tunnel: [w498] -> w486
        tunnel: [w495] -> w485
        tunnel: [w494] -> w484
        tunnel: w483 -> [w493]
        stop <- w506 stop-if-true
        (unwired) 8 ("Number of Objects")
        w515 = u16 1 items=["RGB", "HSL", "HSV", "HSI"] ("Color Mode")
        n129 = flat-sequence {
          tunnel: [w522] -> w501
          tunnel: w500 -> [w520]
          tunnel: w499 -> [w521]
          tunnel: [w521] -> w497
          tunnel: [w520] -> w496
          tunnel: w493 -> [w518]
          tunnel: w501 -> [w533]
          tunnel: [w532] -> w498
          tunnel: w497 -> [w530]
          tunnel: w496 -> [w531]
          tunnel: [w531] -> w495
          tunnel: [w530] -> w494
          frame #0 {
            w523 = 50 ("Motor 1 Encoder Target")
            w527 = i16 100 ("Motor 1 Contant Speed (Degrees per Second)")
            n130 = global read "Global 5.vi" "Count Encode"() -> (w524:dbl)
            n131 = Wait (ms)(milliseconds to wait=u32 500 ("millisecond timer value")) -> ()  [unwired: 1 out]
            n132 = Add(x=w523, y=w524) -> (x+y=w525:dbl)
            n133 = call <vilib>:"TETRIX_Reset_Encoders_myRIO.vi"("myRIO MXP Port A/B"=w520, "Select Encoder"="Encoders 1 and 2", "Controller ID#  (I2C Address)"=w521, "Error/Flow In"=w518) -> ("Error/Flow Out"=w519:errorcluster)  [unwired: 3 in]
            n134 = call <vilib>:"TETRIX_Set_Motor_Target(s)_myRIO.vi"("Motor 2 Encoder Target"=w523, "Motor 1 Encoder Target"=w523, "myRIO MXP Port A/B"=w520, "Controller ID#  (I2C Address)"=w521, "Motor 2 Constant Speed (Degrees per Second)"=w527, "Motor 1 Contant Speed (Degrees per Second)"=w527, "Encoder Units"="Degrees", "Error/Flow In"=w519) -> ("Error/Flow Out"=w522:errorcluster)  [unwired: 1 in]
            n135 = global write "Global 5.vi" "Count Encode"(w525) -> ()
          }
          frame #1 {
            n136 = Wait (ms)(milliseconds to wait=u32 500 ("millisecond timer value")) -> ()  [unwired: 1 out]
            n137 = call <vilib>:"TETRIX_Stop_Motors_myRIO.vi"("myRIO MXP Port A/B"=w531, "Stop Mode"="Brake", "Select Channel"="Both Motors", "Controller ID#  (I2C Address)"=w530, "Error/Flow In"=w533) -> ("Error/Flow Out"=w532:errorcluster)  [unwired: 2 in]
          }
        }
        n138 = call <vilib>:"IMAQdx Snap2.vi"("Image In"=w517, "Session In"=T4 "cam0") -> ("Image Out"=w516:T2)  [unwired: 7 in, 2 out]
        n139 = call "IMAQ ExtractColorPlanes"("Blue or Luma or Val or Inten Plane"=w511, "Color Mode"=w515, "Image Src"=w516) -> ("Blue or Luma or Val or Inten Plane out"=w514:T2)  [unwired: 5 in, 3 out]
        n140 = call "IMAQ Rotate"("Angle (degrees)"=sgl -1.5, "Image Src"=w514) -> ("Image Dst Out"=w507:T2)  [unwired: 8 in, 1 out]
        "Im3" <- w507
        n141 = call "IMAQ Extract 2"("Optional Rectangle"=i32[] [321, 232, 340, 263], "Image Src"=w507) -> ("Image Dst Out"=w510:T2)  [unwired: 8 in, 1 out]
        n142 = property on="Im3" class="ImageControl"() -> ("ROI"=→"ROI 2":T1)  [unwired: 2 in, 2 out]
        n143 = call "IMAQ Count Objects 2"("Settings"=T3 {"Objects"=0, "Threshold"=128, "Reject Border"=FALSE, "Fill Holes"=FALSE, "Min Object Size"=FALSE, "Min Size"=3, "Max Object Size"=FALSE, "Max Size"=100, "Show Search Area"=FALSE, "Show Center"=TRUE, "Show Bounding Box"=TRUE}, "Image"=w510) -> ("Number of Objects"=w505:i32, "Image Out"=→"SecondCount":T2)  [unwired: 5 in, 3 out]
        "Number of Objects 3" <- w505
        n144 = Greater Or Equal?(x=w505, y=2) -> (x >= y?=w506:bool)
      }
      n145 = local write "Status"("IMAQ Start " ("Status")) -> ()
    }
    frame #34 {
      w547 = i16 100 ("Motor 1 Contant Speed (Degrees per Second)")
      n146 = Wait (ms)(milliseconds to wait=u32 4500) -> ()  [unwired: 1 out]
      n147 = call <vilib>:"TETRIX_Reset_Encoders_myRIO.vi"("myRIO MXP Port A/B"=w538, "Select Encoder"="Encoders 1 and 2", "Controller ID#  (I2C Address)"=w537, "Error/Flow In"=w540) -> ("Error/Flow Out"=w542:errorcluster)  [unwired: 3 in]
      n148 = call <vilib>:"TETRIX_Set_Motor_Target(s)_myRIO.vi"("Motor 2 Encoder Target"=-285 ("Motor 1 Encoder Target"), "Motor 1 Encoder Target"=300, "myRIO MXP Port A/B"=w538, "Controller ID#  (I2C Address)"=w537, "Motor 2 Constant Speed (Degrees per Second)"=w547, "Motor 1 Contant Speed (Degrees per Second)"=w547, "Encoder Units"="Degrees", "Error/Flow In"=w542) -> ("Error/Flow Out"=w539:errorcluster)  [unwired: 1 in]
    }
    frame #35 {
      n149 = Wait (ms)(milliseconds to wait=u32 500) -> ()  [unwired: 1 out]
      n150 = call <vilib>:"TETRIX_Stop_Motors_myRIO.vi"("myRIO MXP Port A/B"=w550, "Stop Mode"="Brake", "Select Channel"="Both Motors", "Controller ID#  (I2C Address)"=w551, "Error/Flow In"=w552) -> ("Error/Flow Out"=w549:errorcluster)  [unwired: 2 in]
    }
    frame #36 {
      n151 = call "Shoot.vi"() -> ()  [unwired: 12 in]
      n152 = local write "Back"(FALSE ("Back")) -> ()
      n153 = local write "Status"("Shooting " ("Status")) -> ()
    }
    frame #37 {
      w570 = i16 100 ("Motor 1 Contant Speed (Degrees per Second)")
      n154 = call <vilib>:"TETRIX_Reset_Encoders_myRIO.vi"("myRIO MXP Port A/B"=w563, "Select Encoder"="Encoders 1 and 2", "Controller ID#  (I2C Address)"=w564, "Error/Flow In"=w566) -> ("Error/Flow Out"=w565:errorcluster)  [unwired: 3 in]
      n155 = local write "Status"("Back Home " ("Status")) -> ()
      n156 = Wait (ms)(milliseconds to wait=u32 4500) -> ()  [unwired: 1 out]
      n157 = call <vilib>:"TETRIX_Set_Motor_Target(s)_myRIO.vi"("Motor 2 Encoder Target"=285, "Motor 1 Encoder Target"=-300, "myRIO MXP Port A/B"=w563, "Controller ID#  (I2C Address)"=w564, "Motor 2 Constant Speed (Degrees per Second)"=w570, "Motor 1 Contant Speed (Degrees per Second)"=w570, "Encoder Units"="Degrees", "Error/Flow In"=w565) -> ("Error/Flow Out"=w562:errorcluster)  [unwired: 1 in]
      "Back" <- TRUE ("Back")
    }
    frame #38 {
      n158 = Wait (ms)(milliseconds to wait=u32 500) -> ()  [unwired: 1 out]
      n159 = call <vilib>:"TETRIX_Stop_Motors_myRIO.vi"("myRIO MXP Port A/B"=w575, "Stop Mode"="Brake", "Select Channel"="Both Motors", "Controller ID#  (I2C Address)"=w576, "Error/Flow In"=w577) -> ("Error/Flow Out"=w574:errorcluster)  [unwired: 2 in]
    }
    frame #39 {
      w591 = i16 200 ("Motor 1 Contant Speed (Degrees per Second)")
      n160 = call <vilib>:"TETRIX_Reset_Encoders_myRIO.vi"("myRIO MXP Port A/B"=w582, "Select Encoder"="Encoders 1 and 2", "Controller ID#  (I2C Address)"=w583, "Error/Flow In"=w588) -> ("Error/Flow Out"=w592:errorcluster)  [unwired: 3 in]
      n161 = Wait (ms)(milliseconds to wait=u32 5000) -> ()  [unwired: 1 out]
      n162 = global read "Global 5.vi" "Count Encode"() -> (w587:dbl)
      n163 = local write "Status"("Encode to Home " ("Status")) -> ()
      n164 = Subtract(x=800.0, y=w587) -> (x-y=w585:dbl)
      "x-y" <- w585
      n165 = call <vilib>:"TETRIX_Set_Motor_Target(s)_myRIO.vi"("Motor 2 Encoder Target"=w585, "Motor 1 Encoder Target"=w585, "myRIO MXP Port A/B"=w582, "Controller ID#  (I2C Address)"=w583, "Motor 2 Constant Speed (Degrees per Second)"=w591, "Motor 1 Contant Speed (Degrees per Second)"=w591, "Encoder Units"="Degrees", "Error/Flow In"=w592) -> ("Error/Flow Out"=w584:errorcluster)  [unwired: 1 in]
    }
    frame #40 {
      n166 = call <vilib>:"TETRIX_Stop_Motors_myRIO.vi"("myRIO MXP Port A/B"=w594, "Stop Mode"="Brake", "Select Channel"="Both Motors", "Controller ID#  (I2C Address)"=w595, "Error/Flow In"=w597) -> ("Error/Flow Out"=w596:errorcluster)  [unwired: 2 in]
      n167 = Wait (ms)(milliseconds to wait=u32 500) -> ()  [unwired: 1 out]
    }
    frame #41 {
      w609 = i16 100 ("Motor 1 Contant Speed (Degrees per Second)")
      n168 = call <vilib>:"TETRIX_Reset_Encoders_myRIO.vi"("myRIO MXP Port A/B"=w603, "Select Encoder"="Encoders 1 and 2", "Controller ID#  (I2C Address)"=w604, "Error/Flow In"=w602) -> ("Error/Flow Out"=w606:errorcluster)  [unwired: 3 in]
      n169 = local write "Status"("Turning" ("Status")) -> ()
      n170 = Wait (ms)(milliseconds to wait=u32 4500) -> ()  [unwired: 1 out]
      n171 = call <vilib>:"TETRIX_Set_Motor_Target(s)_myRIO.vi"("Motor 2 Encoder Target"=290, "Motor 1 Encoder Target"=-295, "myRIO MXP Port A/B"=w603, "Controller ID#  (I2C Address)"=w604, "Motor 2 Constant Speed (Degrees per Second)"=w609, "Motor 1 Contant Speed (Degrees per Second)"=w609, "Encoder Units"="Degrees", "Error/Flow In"=w606) -> ()  [unwired: 1 in, 1 out]
    }
    frame #42 {
      n172 = call <vilib>:"TETRIX_Stop_Motors_myRIO.vi"("myRIO MXP Port A/B"=w614, "Stop Mode"="Brake", "Select Channel"="Both Motors", "Controller ID#  (I2C Address)"=w615, "Error/Flow In"=w613) -> ("Error/Flow Out"=w612:errorcluster)  [unwired: 2 in]
      n173 = Wait (ms)(milliseconds to wait=u32 500) -> ()  [unwired: 1 out]
    }
    frame #43 {
      w627 = i16 200 ("Motor 1 Contant Speed (Degrees per Second)")
      n174 = call <vilib>:"TETRIX_Reset_Encoders_myRIO.vi"("myRIO MXP Port A/B"=w620, "Select Encoder"="Encoders 1 and 2", "Controller ID#  (I2C Address)"=w621, "Error/Flow In"=w623) -> ("Error/Flow Out"=w622:errorcluster)  [unwired: 3 in]
      n175 = Wait (ms)(milliseconds to wait=u32 8000) -> ()  [unwired: 1 out]
      n176 = call <vilib>:"TETRIX_Set_Motor_Target(s)_myRIO.vi"("Motor 2 Encoder Target"=900, "Motor 1 Encoder Target"=900, "myRIO MXP Port A/B"=w620, "Controller ID#  (I2C Address)"=w621, "Motor 2 Constant Speed (Degrees per Second)"=w627, "Motor 1 Contant Speed (Degrees per Second)"=w627, "Encoder Units"="Degrees", "Error/Flow In"=w622) -> ("Error/Flow Out"=w619:errorcluster)  [unwired: 1 in]
    }
    frame #44 {
      n177 = local write "Status"("Welcome Home" ("Status")) -> ()
      n178 = Wait (ms)(milliseconds to wait=u32 500) -> ()  [unwired: 1 out]
      n179 = call <vilib>:"TETRIX_Stop_Motors_myRIO.vi"("myRIO MXP Port A/B"=w632, "Stop Mode"="Brake", "Select Channel"="Both Motors", "Controller ID#  (I2C Address)"=w633, "Error/Flow In"=w631) -> ()  [unwired: 2 in, 1 out]
    }
  }
